vi "ErrCheck_X mirror speed within limits.vi"(8 "Error In":errorcluster, 11 "Settings ArrayIN":T1[](array[typedef])) -> (0 "Error Out":errorcluster, 1 "Not Enough Variables (Warning)?":bool, 2 "Error/Warning Message":string, 3 "Speed  out of Limits?":bool)   [LabVIEW 2012]
doc: "SciScan 1.2 160622"
uses:
  MacroGUI Module/Custom Controls and Typedefs/GFG Variable for IO.ctl
  Custom Controls/MAIN Image panel tab Control type def.ctl
  GFG/GFGnumericGet.vi
  GFG/GFG library.lvlib
  GFG/GFGbooleanGet.vi
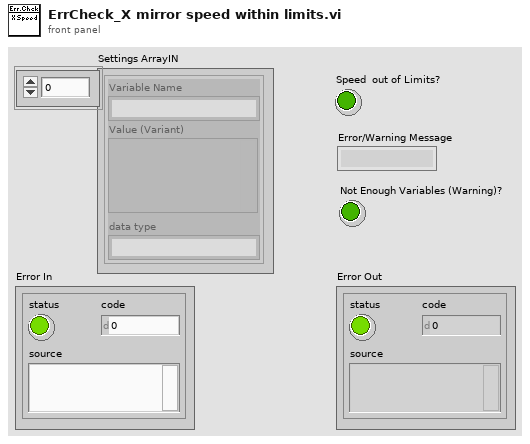
[diagram p1: front panel]
types:
  T1 = typedef "GFG Variable for IO.ctl" = cluster{"Variable Name":string, "Value (Variant)":variant, "data type":string}
  T2 = typedef "MAIN Image panel tab Control type def.ctl" = enum32{"Channel 1", "Channel 2", "Channel 3", "Channel 4", "all channels", "RGB overlay", "ROI", "arbitrary line scan"}
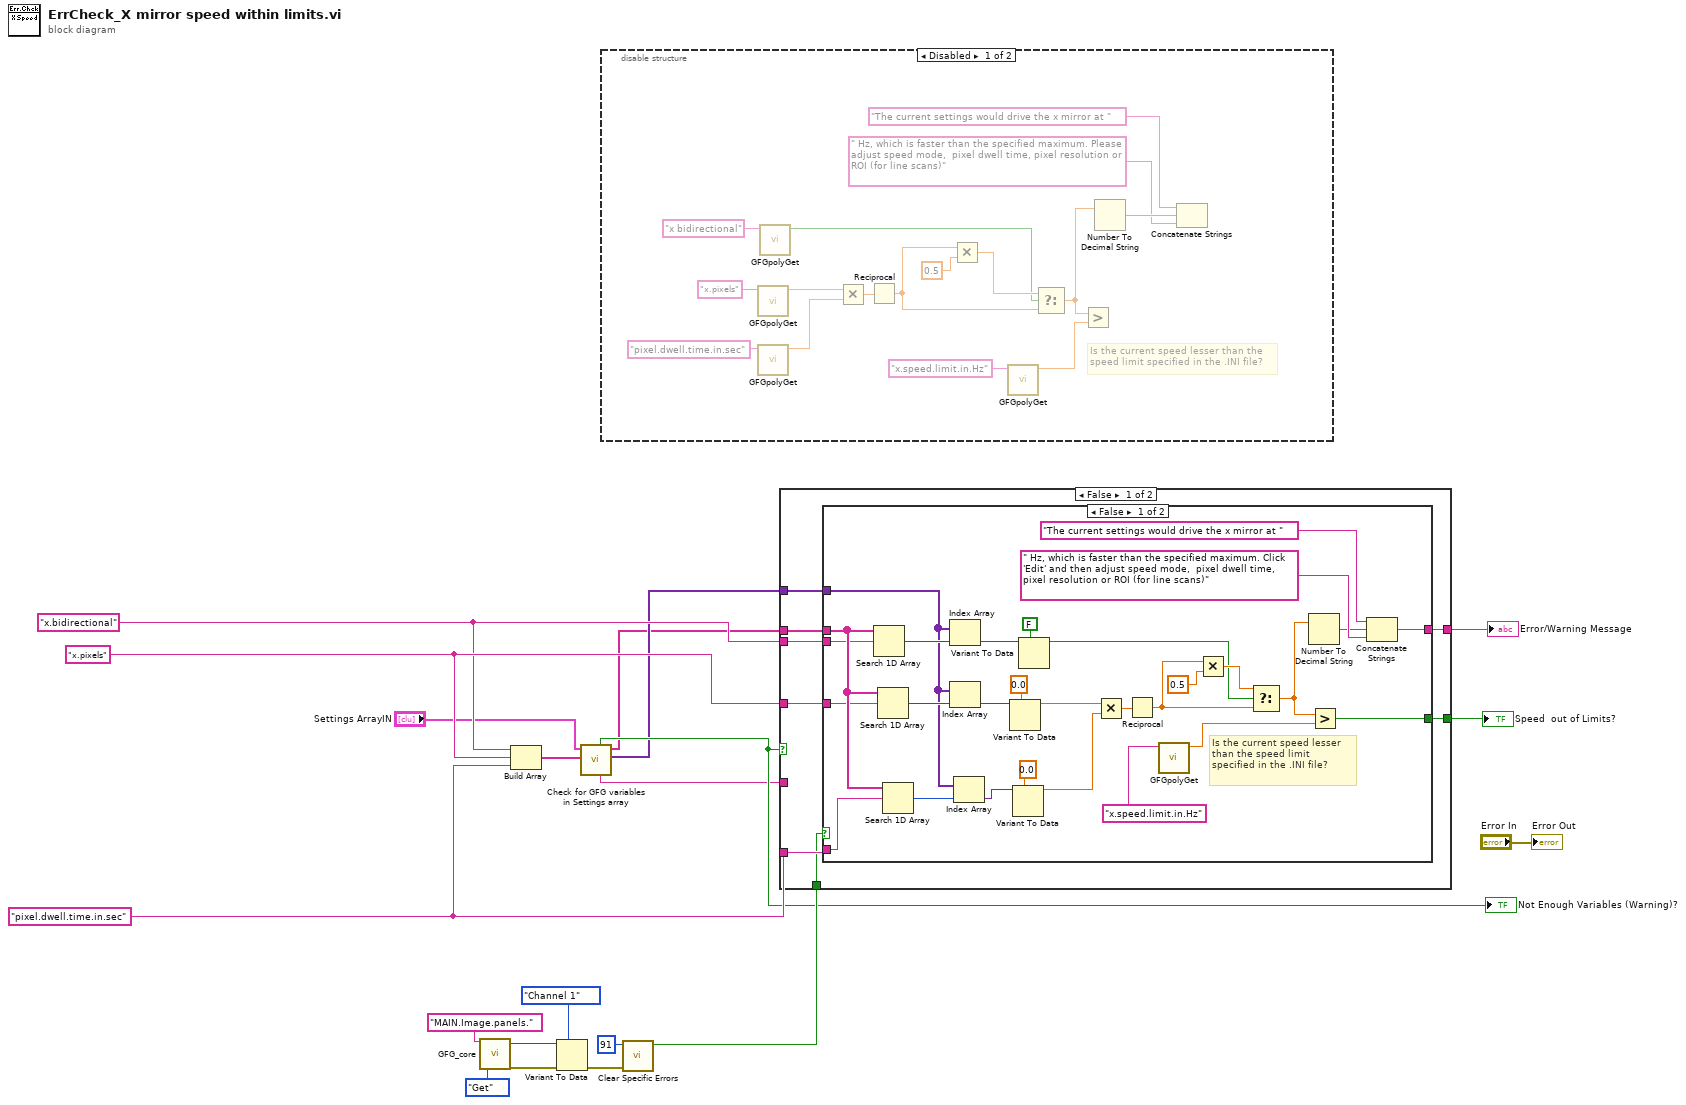
[diagram p0: block diagram]
diagram:
  w17 = "x.bidirectional" ("Variable Name in")
  w18 = "x.pixels" ("Variable Name in")
  w19 = "pixel.dwell.time.in.sec" ("Variable Name in")
  n1 = call "GFG_core.vi"("Variable Name in"="MAIN.Image.panels.", "Action"=enum16{"Init", "Set", "Get", "Clear"}."Get") -> ("Variant Out"=w12:variant, "error out"=w9:errorcluster)  [unwired: 11 in, 5 out]
  n2 = Build Array(w17, w18, w19) -> (w1:string[])
  n3 = Variant To Data(error in=w9, type=MAIN_Image_panel_tab_Control_type_def."Channel 1" ("MAIN Image panels"), Variant=w12) -> (error out=w13:errorcluster)  [unwired: 1 out]
  n4 = call "Check for GFG variables in Settings array.vi"("GFG variables to search"=w1, "Settings ArrayIN"="Settings ArrayIN") -> ("GFG variant values (those found)"=w4:variant[], "GFG variables found"=w3:string[], "Error Message (list of variables not found)"=w5:string, "Any Not Found?"=w6:bool)  [unwired: 4 in, 2 out]
  "Not Enough Variables (Warning)?" <- w6
  n5 = disable-structure shown="Disabled" {
    frame Disabled {
      # "Is the current speed lesser than the\nspeed limit specified in the .INI file?"
      n6 = call-poly "GFGpolyGet.vi"("Variable Name in"="x.pixels") -> ("Numeric"=w26:dbl)  [unwired: 8 in, 2 out]
      n7 = call-poly "GFGpolyGet.vi"("Variable Name in"="pixel.dwell.time.in.sec") -> ("Numeric"=w25:dbl)  [unwired: 8 in, 2 out]
      n8 = call-poly "GFGpolyGet.vi"("Variable Name in"="x bidirectional") -> ("Boolean Value OUT"=w27:bool)  [unwired: 9 in, 1 out]
      n9 = Multiply(x=w26, y=w25) -> (x*y=w28:dbl)
      n10 = Reciprocal(x=w28) -> (1/x=w29:dbl)
      n11 = Multiply(x=w29, y=0.5) -> (x*y=w30:dbl)
      n12 = call-poly "GFGpolyGet.vi"("Variable Name in"="x.speed.limit.in.Hz") -> ("Numeric"=w33:dbl)  [unwired: 8 in, 2 out]
      n13 = Select(t=w30, s=w27, f=w29) -> (s? t:f=w21:dbl)
      n14 = Greater?(x=w21, y=w33) -> ()  [unwired: 1 out]
      n15 = Number To Decimal String(number=w21) -> (decimal integer string=w23:string)  [unwired: 1 in]
      n16 = Concatenate Strings("The current settings would drive the x mirror at " ("message"), w23, " Hz, which is faster than the specified maximum. Please adjust speed mode,  pixel dwell time, pixel resolution or ROI (for line scans)" ("string")) -> ()  [unwired: 1 out]
    }
    frame Enabled {
    }
  }
  n17 = call "Clear Specific Errors.vi"("Error In"=w13, "Error number In"=91) -> ("Error Cleared?"=w7:bool)  [unwired: 8 in, 1 out]
  n18 = case shown="False" w6 {
    tunnel: [w39 w74] -> w16
    tunnel: w3 -> [w44 _]
    tunnel: w4 -> [w43 _]
    tunnel: w19 -> [w42 _]
    tunnel: w18 -> [w41 _]
    tunnel: w17 -> [w40 _]
    tunnel: [w38 _] -> w15
    tunnel: w7 -> [w37 _]
    tunnel: w5 -> [_ w74]
    frame False {
      n19 = case shown="False" w37 {
        tunnel: w44 -> [w59 _]
        tunnel: w43 -> [w54 _]
        tunnel: w42 -> [w49 _]
        tunnel: w41 -> [w48 _]
        tunnel: w40 -> [w47 _]
        tunnel: [w46 _] -> w39
        tunnel: [w45 _] -> w38
        frame False {
          # "Is the current speed lesser than the speed limit specified in the .INI file?"
          n20 = Search 1D Array(1D array=w59, element=w47) -> (index of element=w63:i32)  [unwired: 1 in]
          n21 = Search 1D Array(1D array=w59, element=w48) -> (index of element=w58:i32)  [unwired: 1 in]
          n22 = Search 1D Array(1D array=w59, element=w49) -> (index of element=w53:i32)  [unwired: 1 in]
          n23 = Index Array(array=w54, index=w63) -> (element=w62:variant)
          n24 = Index Array(array=w54, index=w58) -> (element=w57:variant)
          n25 = Index Array(array=w54, index=w53) -> (element=w52:variant)
          n26 = Variant To Data(type=0.0 ("y"), Variant=w57) -> (data=w51:dbl)  [unwired: 1 in, 1 out]
          n27 = Variant To Data(type=0.0 ("y"), Variant=w52) -> (data=w50:dbl)  [unwired: 1 in, 1 out]
          n28 = Variant To Data(type=FALSE, Variant=w62) -> (data=w60:bool)  [unwired: 1 in, 1 out]
          n29 = Multiply(x=w51, y=w50) -> (x*y=w69:dbl)
          n30 = Reciprocal(x=w69) -> (1/x=w68:dbl)
          n31 = call-poly "GFGpolyGet.vi"("Variable Name in"="x.speed.limit.in.Hz") -> ("Numeric"=w64:dbl)  [unwired: 8 in, 2 out]
          n32 = Multiply(x=w68, y=0.5) -> (x*y=w67:dbl)
          n33 = Select(t=w67, s=w60, f=w68) -> (s? t:f=w73:dbl)
          n34 = Number To Decimal String(number=w73) -> (decimal integer string=w71:string)  [unwired: 1 in]
          n35 = Greater?(x=w73, y=w64) -> (0:w45:bool)
          n36 = Concatenate Strings("The current settings would drive the x mirror at " ("message"), w71, " Hz, which is faster than the specified maximum. Click 'Edit' and then adjust speed mode,  pixel dwell time, pixel resolution or ROI (for line scans)" ("string")) -> (w46:string)
        }
        frame True {
          # "Donot run the speed check for RESO system"
        }
      }
    }
    frame True {
    }
  }
  "Speed  out of Limits?" <- w15
  "Error/Warning Message" <- w16
  "Error Out" <- "Error In"
